vi "TESTnew-PI-2.vi"() -> ()   [LabVIEW 2014]
panel:
  in  "Rec. table":i32
  in  "Value":string[](array[string])
  in  "DataRecorderTable":i32[](array[numeric])
  in  "Rec. table IDs":i32[](array[numeric])
  in  "Nmax":i32=1024
  in  "N":i32=100
  out "Data":dbl[][](array[numeric]) format="%.6f"
  out "Names":string[](array[string])
  out "Waveform Graph":dbl[](graph)
  in  "Source ID":string
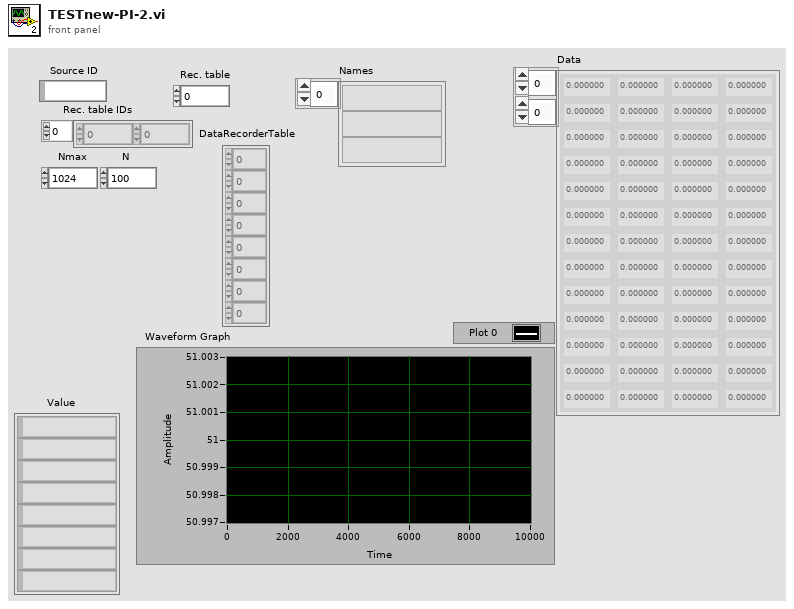
[diagram p1: front panel]
types:
  T1 = enum16{"default", "changing target position", "external trigger", "immediately"}
  T2 = enum16{"Target position", "Current position", "position error"}
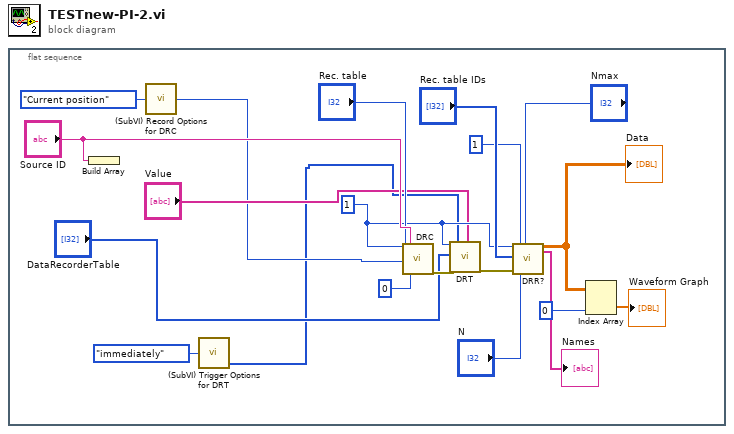
[diagram p0: block diagram]
diagram:
  n1 = flat-sequence {
    frame #0 {
      w8 = 1 ("System no.")
      n2 = Build Array("Source ID") -> ()  [unwired: 1 out]
      n3 = call "(SubVI) Record Options for DRC.vi"("Enum"=T2."Current position") -> ("Record options"=w3:i32)  [unwired: 4 in]
      n4 = call "(SubVI) Trigger Options for DRT.vi"("Enum"=T1."immediately") -> ("trigger source array for DRT"=w1:i32[])  [unwired: 3 in, 1 out]
      n5 = call "DRC.vi"("System no."=w8, "Rec. table"="Rec. table", "Rec. option"=w3, "Source ID"="Source ID", "Trigger option"=0) -> ("error out"=w9:errorcluster)  [unwired: 1 in, 13 out]
      n6 = call "DRT.vi"("System no."=w8, "DataRecorderTable"="DataRecorderTable", "error in"=w9, "Trigger source"=w1, "Value"="Value") -> ("error out"=w7:errorcluster)  [unwired: 14 out]
      n7 = call "DRR?.vi"("System no."=w8, "Rec. table IDs"="Rec. table IDs", "error in"=w7, "Xo"=1, "N"="N", "Nmax"="Nmax") -> ("Data"=w16:dbl[][], "Names"=→"Names":string[])  [unwired: 2 in, 10 out]
      "Data" <- w16
      n8 = Index Array(array=w16, index (col)=0 ("disabled index (col)")) -> (element=→"Waveform Graph":dbl[])  [unwired: 1 in]
    }
  }
